vi "Write SP REMOTE Comm Parameters.vi"(8 "error in (no error)":errorcluster, 10 "SP REMOTE Comm Parameters":T1={"SemiProbe VISA"="", "write delay(ms)"=500, "buffer is full loop multiplicity"=10, "read threshold check rate (ms)"=50}, 11 "SemiProbe in":refnum<class "SemiProbe.lvclass">) -> (0 "error out":errorcluster, 3 "SemiProbe out":refnum<class "SemiProbe.lvclass">)   [LabVIEW 2013, in "SemiProbe.lvclass"]
uses:
  SemiProbe.lvclass
  SemiProbe.lvclass/SemiProbe.ctl
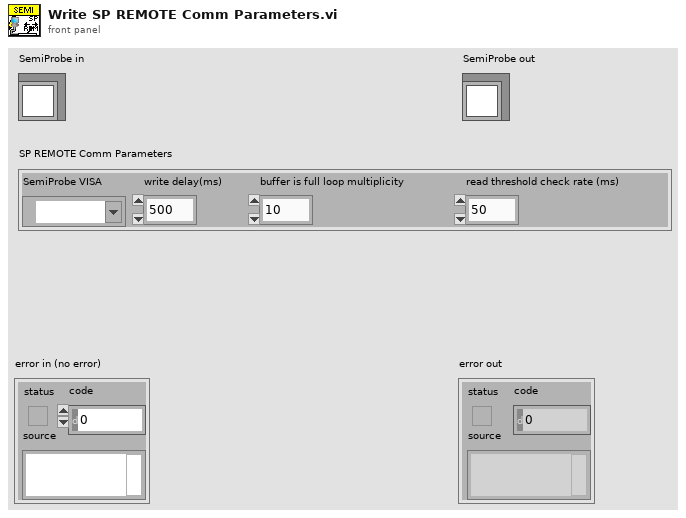
[diagram p1: front panel]
types:
  T1 = cluster{"SemiProbe VISA":refnum<visa-resource-name>, "write delay(ms)":i32, "buffer is full loop multiplicity":i32, "read threshold check rate (ms)":u32}
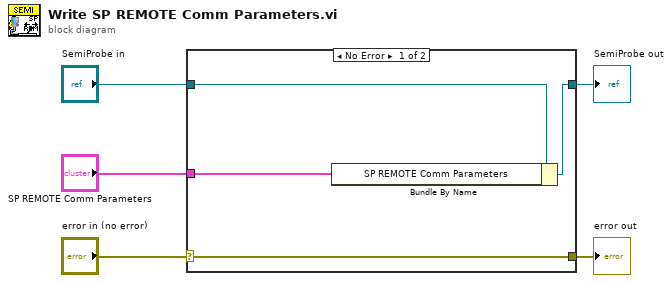
[diagram p0: block diagram]
diagram:
  n1 = case shown="No Error" "error in (no error)" {
    selector: "error in (no error)" -> [w9 w10]
    tunnel: [w9 w10] -> w4
    tunnel: [w7 w11] -> w2
    tunnel: "SemiProbe in" -> [w8 w11]
    tunnel: "SP REMOTE Comm Parameters" -> [w6 _]
    frame No Error {
      n2 = Bundle By Name(cluster=w8, "SP REMOTE Comm Parameters"=w6) -> (w7:refnum<class "SemiProbe.lvclass">)
    }
    frame Error {
    }
  }
  "error out" <- w4
  "SemiProbe out" <- w2
